vi "flow-builder-nutrition-dose.vi"(7 "Proc Name (empty: bypass logging)":string="UNIT%d", 9 "Unit Index":i32, 10 "Digital Timeout":u16, 11 "OUTPUT(+AUX)":string[](array[string])) -> (0 "error out":errorcluster, 3 "intructions out":variant[](array[variant]))   [LabVIEW 2024]
uses:
  controls/UiStepBuilder.ctl
  controls/type.step-builder.ctl
  build.flowToVarient.vi
  Polymorphics/variantCtrl.polymorphic.vi
  Polymorphics/variantCtrlStepFunction.vi
  Polymorphics/variantCtrlSetpoint.vi
  Polymorphics/variantCtrlString.vi
  proc.util.enumToStrStepVar.vi
  util.DelimitedStringFromArray.vi
  Polymorphics/variantCtrlNumber.vi
  util.DelimitedStringToArray.vi
  proc.util.validateParamExist.vi
  <vilib>/Utility/error.llb/Clear Errors.vi
  <vilib>/Utility/error.llb/Trim Whitespace.vi
  <vilib>/Utility/error.llb/Trim Whitespace One-Sided.vi
  build.elementToParamString.vi
  util.error.create.vi
  Polymorphics/variantCtrlStepPointer.vi
  Polymorphics/variantCtrlStepUserMessage.vi
  Polymorphics/variantCtrlStepPath.vi
panel:
  out "Flow":T1[](array[typedef])
  # "UNIT-DOSE(UNIT,OUTPUT, TIMEOUT)"
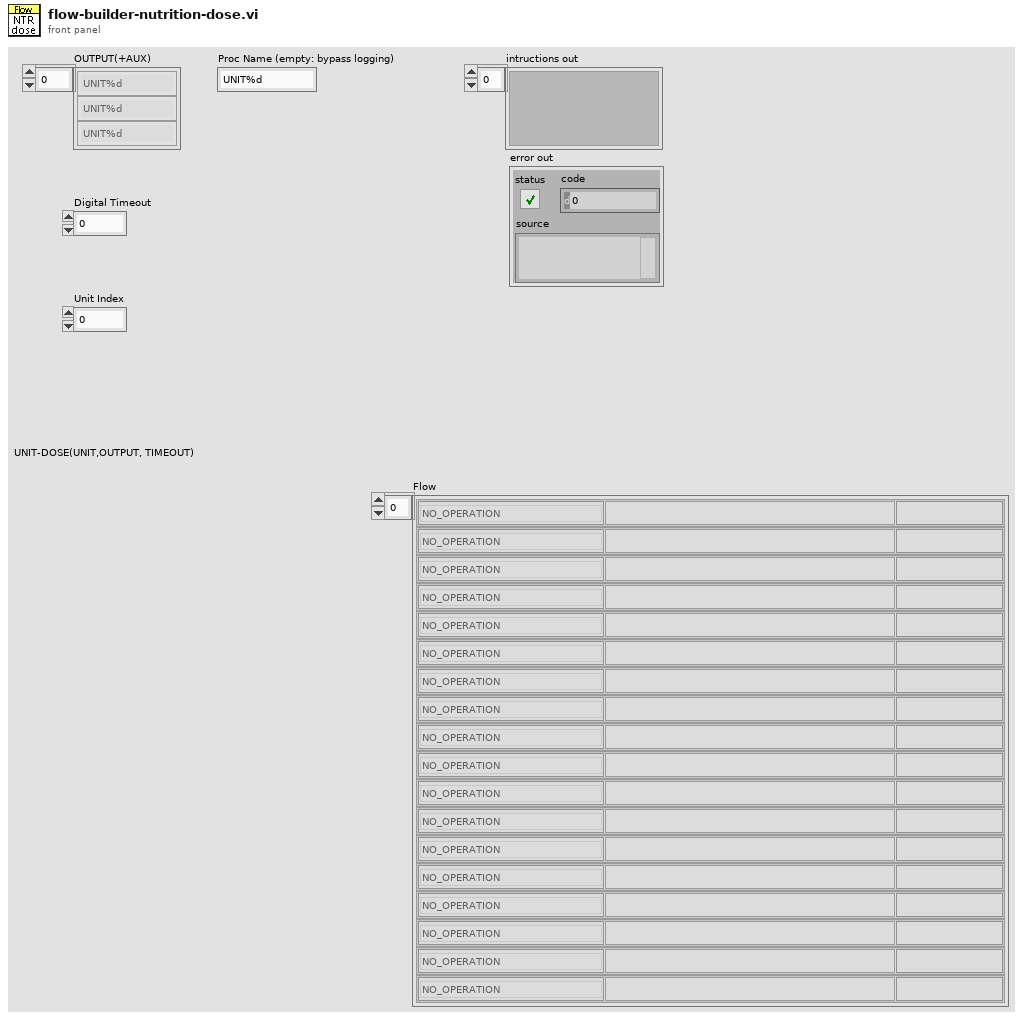
[diagram p1: front panel]
types:
  T1 = typedef "UiStepBuilder.ctl" = cluster{"Step Function":T2, "ParamString":string, "Step Label":string}
  T2 = typedef "type.step-builder.ctl" = enum16{"NO_OPERATION", "DELAY-JUMP", "DELAY", "JUMP", "COMPLETE", "SCHEDULER", "IRR-CHECK", "UNIT-CHECK", "UNIT-SAMPLE", "UNIT-DOSE", "LOG-REPORT", "LOG-MESSAGE", "IO-READ", "IO-READ-MANY", "IO-WRITE", "IO-COMPARE-OUT", "IO-COMPARE-IN", "PROC-START", "PROC-STOP", "PROC-LOAD", "PROC-IS-COMPLETED", "RECORD-MOVE", "GET-RH", "GET-UV", "GET-WD", "GET-WS", "OCS-CHECK", "OCS-RECORD"}
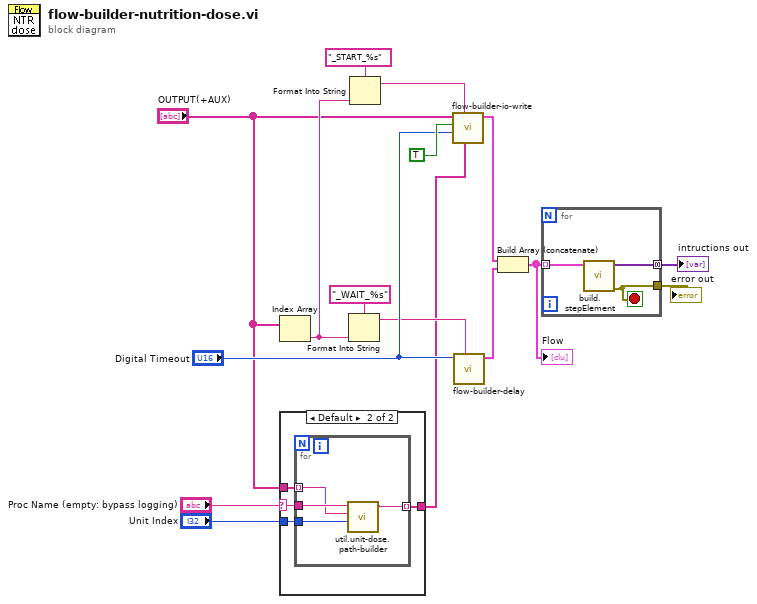
[diagram p0: block diagram]
diagram:
  n1 = Index Array(array="OUTPUT(+AUX)") -> (element=w7:string)  [unwired: 1 in]
  n2 = case shown="Default" "Proc Name (empty: bypass logging)" {
    selector: "Proc Name (empty: bypass logging)" -> [_ w19]
    tunnel: "OUTPUT(+AUX)" -> [_ w20]
    tunnel: "Unit Index" -> [_ w18]
    tunnel: [_ w17] -> w2
    frame "False" {
    }
    frame Default {
      n3 = for {
        tunnel: w20 -> [w23] mode=indexing
        tunnel: w19 -> [w24]
        tunnel: w18 -> [w22]
        tunnel: [w21] -> w17 mode=indexing
        n4 = call "util.unit-dose.path-builder.vi"("Unit Index"=w22, "Input"=w23, "Proc Name"=w24) -> ("\\NUTRITION\\ORP\\ORP_U1_2024-08-16.*"=w21:string)  [unwired: 8 in]
      }
    }
  }
  n5 = Format Into String(format string="_WAIT_%s", w7) -> (resulting string=w9:string)  [unwired: 2 in, 1 out]
  n6 = Format Into String(format string="_START_%s", w7) -> (resulting string=w6:string)  [unwired: 2 in, 1 out]
  n7 = call "flow-builder-io-write.vi"("filenames.*"=w2, "Step Name"=w6, "Digital Timeout"="Digital Timeout", "Value in"=TRUE, "Dout+AUX"="OUTPUT(+AUX)") -> ("Flow out"=w13:T1[])  [unwired: 6 in]
  n8 = call "flow-builder-delay.vi"("Step Label"=w9, "Delay [s]"="Digital Timeout") -> ("Step Element"=w12:T1)  [unwired: 9 in]
  n9 = Build Array (concatenate)(w13, w12) -> (w11:T1[])
  "Flow" <- w11
  n10 = for {
    tunnel: w11 -> [w27] mode=indexing
    tunnel: [w26] -> w16 mode=concatenating
    tunnel: [w25] -> w1
    stop <- w25 stop-if-true
    n11 = call "build.stepElement.vi"("Step in"=w27) -> ("error out"=w25:errorcluster, "steps out"=w26:variant[])  [unwired: 9 in]
  }
  "intructions out" <- w16
  "error out" <- w1
